vi "fgv_procon-q.vi"(7 "cmd 2":T1, 8 "error in":errorcluster, 10 "hw lists":T2, 11 "data":T3=enum."stop") -> (0 "error out":errorcluster, 2 "q-refs":refnum<queue>[](array[refnum]), 3 "ref":refnum<queue>)   [LabVIEW 2021]
uses:
  ctrl/q-data_run-check-stop.ctl
  Karnavi_MultiSerial/VIs/_ctrl/run-check-stop.ctl
  ctrl/hw-lists.ctl
  ctrl/create-rw-close.ctl
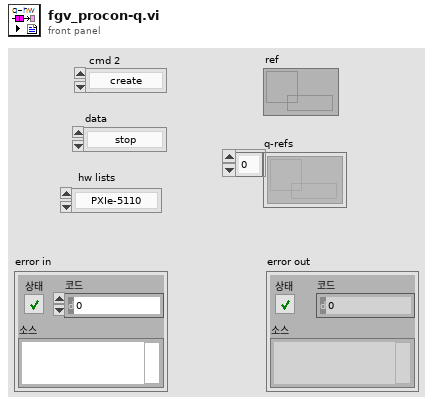
[diagram p1: front panel]
types:
  T1 = typedef "create-rw-close.ctl" = enum16{"create", "read", "write", "close"}
  T2 = typedef "hw-lists.ctl" = enum16{"PXIe-5110", "PXIe-5413", "PXIe-2530", "DS1202"}
  T3 = typedef "q-data_run-check-stop.ctl" = enum16{"run", "check", "stop"}
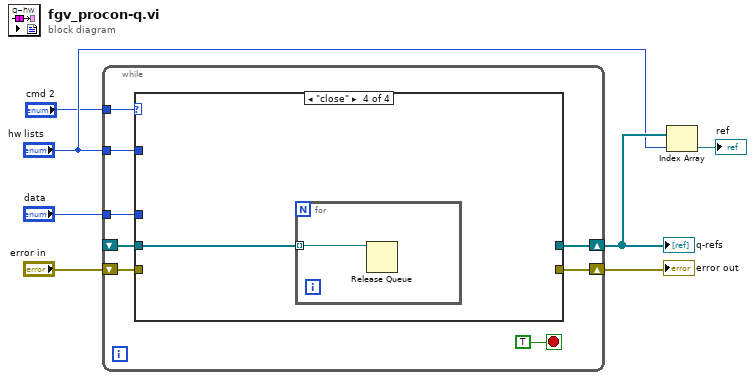
[diagram p0: block diagram]
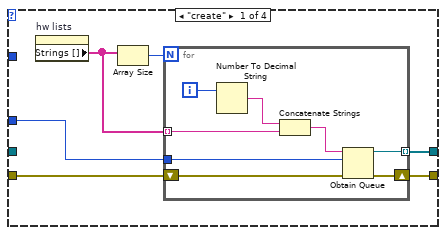
[diagram p2: hidden frame]
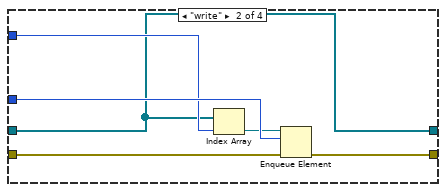
[diagram p3: hidden frame]
diagram:
  n1 = while {
    tunnel: "cmd 2" -> [w15]
    shift-right: [w11] -> w4
    shift-left: _ -> [w10]
    shift-right: [w12] -> w7
    shift-left: "error in" -> [w13]
    tunnel: "data" -> [w9]
    tunnel: "hw lists" -> [w8]
    stop <- TRUE stop-if-true
    n2 = case shown="\"close\"" w15 {
      tunnel: w13 -> [w21 w35 w36 _]
      tunnel: [w20 w34 w36 _] -> w12
      tunnel: [w19 w30 w37 _] -> w11
      tunnel: w10 -> [_ w30 w37 w38]
      tunnel: w9 -> [w18 w33 _ _]
      tunnel: w8 -> [_ w32 _ _]
      frame "create" {
        n3 = property on="hw lists" class="Enum (strict)"() -> ("Strings []"=w16:string[])  [unwired: 2 in, 2 out]
        n4 = Array Size(array=w16) -> (size(s)=w17:i32)
        n5 = for {
          N: w17 -> [_]
          tunnel: [w27] -> w19 mode=indexing
          tunnel: w18 -> [w26]
          shift-right: [w28] -> w20
          shift-left: w21 -> [w29]
          tunnel: w16 -> [w23] mode=indexing
          i -> [w25]
          n6 = Number To Decimal String(number=w25) -> (decimal integer string=w24:string)  [unwired: 1 in]
          n7 = Concatenate Strings(w24, w23) -> (w22:string)
          n8 = Obtain Queue(name (unnamed)=w22, element data type=w26, error in (no error)=w29) -> (queue out=w27:refnum<queue>, error out=w28:errorcluster)  [unwired: 2 in, 1 out]
        }
      }
      frame "write" {
        n9 = Index Array(array=w30, index=w32) -> (element=w31:refnum<queue>)
        n10 = Enqueue Element(queue=w31, element=w33, error in (no error)=w35) -> (error out=w34:errorcluster)  [unwired: 1 in, 2 out]
      }
      frame "read", Default {
      }
      frame "close" {
        n11 = for {
          tunnel: w38 -> [w39] mode=indexing
          n12 = Release Queue(queue=w39) -> ()  [unwired: 2 in, 3 out]
        }
      }
    }
  }
  "error out" <- w7
  "q-refs" <- w4
  n13 = Index Array(array=w4, index="hw lists") -> (element=→"ref":refnum<queue>)
